vi "testEmptyDataSet.vi"() -> ()   [LabVIEW 2019, in "TestCaseTest.lvlib" / "Theory.lvlib"]
uses:
  Theory.lvlib
  TestCase/Theory/Theory.lvclass
  Support/Support.lvlib
  Assertion/Assertion.lvlib
panel:
  out "error out":errorcluster
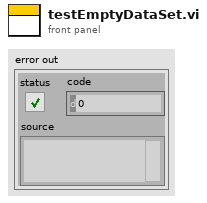
[diagram p1: front panel]
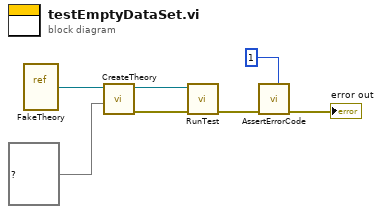
[diagram p0: block diagram]
diagram:
  n1 = vi-ref "FakeTheory.vi"() -> (w1:refnum<vi>)
  n2 = call "CreateTheory.vi"("Control Data"=map{string, variant} {}, "VI Refnum"=w1) -> ("error out"=w6:errorcluster, "Theory"=w7:refnum<class "Theory.lvclass">)  [unwired: 8 in]
  n3 = call-dynamic "RunTest.vi"("error in (no error)"=w6, "Theory in"=w7) -> ("error out"=w5:errorcluster)  [unwired: 8 in, 1 out]
  n4 = call "AssertErrorCode.vi"("Expected"=1, "error in (no error)"=w5) -> ("error out"=→"error out":errorcluster)  [unwired: 9 in]
